vi "chkEmptyWrite.vi"(8 "error in (no error)":errorcluster, 10 "Select Macro Function":T1(ring), 11 "Write Data (HEX)":string) -> (0 "error out":errorcluster, 3 "Write Data Out":string)   [LabVIEW 2019]
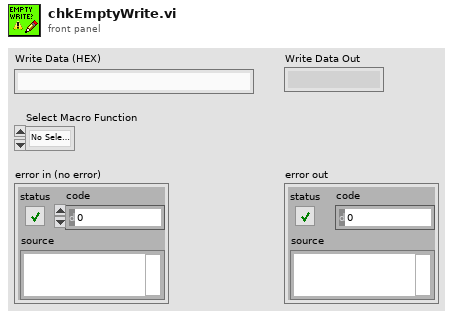
[diagram p1: front panel]
types:
  T1 = enum32{"No Selection", "WRITE", "READ", "WRITE -> READ", "READ -> WRITE -> READ", "ON/OFF", "NO ARGS"}
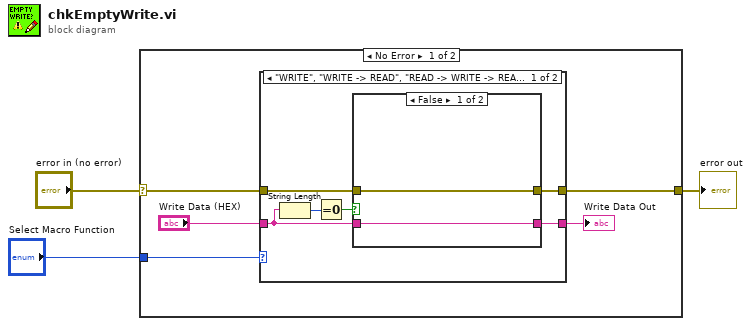
[diagram p0: block diagram]
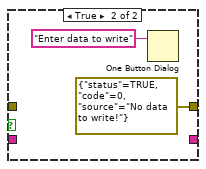
[diagram p2: hidden frame]
diagram:
  n1 = case shown="No Error" "error in (no error)" {
    selector: "error in (no error)" -> [w4 w20]
    tunnel: [w6 w20] -> w3
    tunnel: "Select Macro Function" -> [w5 _]
    frame No Error {
      n2 = case shown="\"WRITE\", \"WRITE -> READ\", \"READ -> WRITE -> READ\"" w5 {
        tunnel: w4 -> [w13 w19]
        tunnel: [w12 _] -> w8
        tunnel: [w11 w19] -> w6
        tunnel: "Write Data (HEX)" -> [w10 _]
        frame "WRITE", "WRITE -> READ", "READ -> WRITE -> READ" {
          n3 = String Length(string=w10) -> (length=w9:i32)
          n4 = Equal To 0?(x=w9) -> (x = 0?=w14:bool)
          n5 = case shown="False" w14 {
            tunnel: w10 -> [w15 _]
            tunnel: [w16 errorcluster {"status"=TRUE, "code"=0, "source"="No data to write!"} ("error constant")] -> w11
            tunnel: w13 -> [w16 _]
            tunnel: [w15 _] -> w12
            frame False {
            }
            frame True {
              n6 = One Button Dialog(message="Enter data to write") -> ()  [unwired: 1 in, 1 out]
            }
          }
        }
        frame "READ", Default {
        }
      }
      "Write Data Out" <- w8
    }
    frame Error {
    }
  }
  "error out" <- w3
